vi "EOL NVH Status HMI.vi"() -> ()   [LabVIEW 2018]
panel:
  out "Motion Type":string
  in  "停止":bool
  out "NVH Status":string
  out "OUTPUT":bool[](array[boolean])
  out "INPUT":bool[](array[boolean])
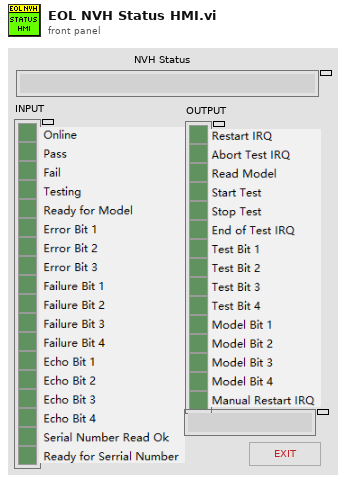
[diagram p1: front panel]
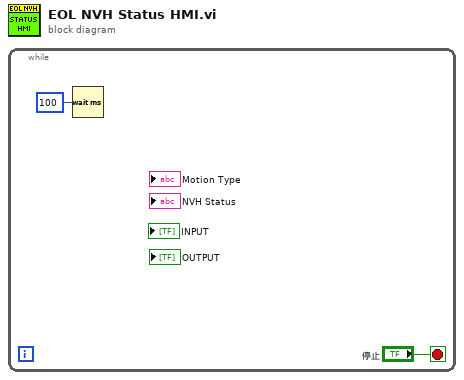
[diagram p0: block diagram]
diagram:
  n1 = while {
    stop <- "停止" stop-if-true
    n2 = Wait (ms)(milliseconds to wait=u32 100 ("等待时间（毫秒）")) -> ()  [unwired: 1 out]
  }
